vi "Generate write queue item.vi"(8 "error in (no error)":errorcluster, 10 "Request ID":u64, 11 "wamplv.lvlib:CallRequest (JSON).lvclass":refnum<class "CallRequest (JSON).lvclass">) -> (0 "error out":errorcluster, 3 "Write queue item":T1)   [LabVIEW 2020, in "wamplv.lvlib" / "CallRequest (JSON).lvclass"]
uses:
  CallRequest (JSON).lvclass
  WAMP Client/Private/TypeDef/Write queue item.ctl
  TypeDefs/Transport type.ctl
  TypeDefs/WAMP Message Codes.ctl
  CallRequest (JSON).lvclass/CallRequest (JSON).ctl
  8d3f56c2-5707-484f-8241-7d0afc6948b6.vi
  wamplv.lvlib
  Utils/Utils.lvclass
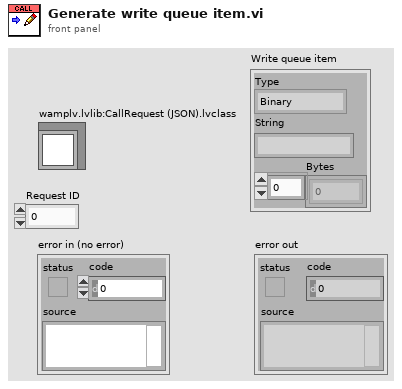
[diagram p1: front panel]
types:
  T1 = typedef "wamplv.lvlib/Write queue item.ctl" = cluster{"Type":T2, "String":string, "Bytes":u8[]}
  T2 = typedef "wamplv.lvlib/Transport type.ctl" = enum16{"Binary", "Text"}
  T3 = typedef "wamplv.lvlib/WAMP Message Codes.ctl" = enum8{"HELLO", "WELCOME", "CHALLENGE", "AUTHENTICATE", "ABORT", "GOODBYE", "ERROR", "PUBLISH", "PUBLISHED", "SUBSCRIBE", "SUBSCRIBED", "UNSUBSCRIBE", "UNSUBSCRIBED", "EVENT", "CALL", "RESULT", "REGISTER", "REGISTERED", "UNREGISTER", "UNREGISTERED", "INVOCATION", "YIELD"}
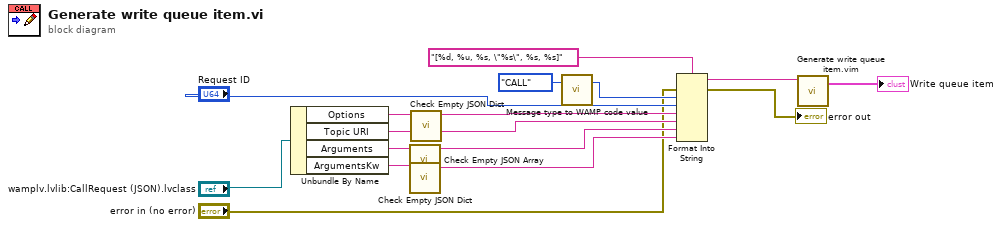
[diagram p0: block diagram]
diagram:
  n1 = Unbundle By Name("wamplv.lvlib:CallRequest (JSON).lvclass") -> ("Options"=w11:string, "Topic URI"=w14:string, "Arguments"=w15:string, "ArgumentsKw"=w13:string)
  n2 = call "Check Empty JSON Array.vi"("JSON in"=w15) -> ("JSON out"=w16:string)  [unwired: 10 in]
  n3 = call "Check Empty JSON Dict.vi"("JSON in"=w13) -> ("JSON out"=w12:string)  [unwired: 10 in]
  n4 = call "Check Empty JSON Dict.vi"("JSON in"=w11) -> ("JSON out"=w10:string)  [unwired: 10 in]
  n5 = call "Message type to WAMP code value.vi"("Message Type"=WAMP_Message_Codes."CALL") -> ("WAMP Numeric value"=w3:u8)  [unwired: 2 in]
  n6 = Format Into String(format string="[%d, %u, %s, \"%s\", %s, %s]" ("element"), error in="error in (no error)", w3, "Request ID", w10, w14, w16, w12) -> (resulting string=w7:string, error out=→"error out":errorcluster)  [unwired: 1 in]
  n7 = call "Generate write queue item.vim"("Input"=w7) -> ("Ouput"=→"Write queue item":T1)  [unwired: 2 in]
